vi "Read UDP.vi"(8 "error in (no error)":errorcluster, 11 "Telnet V2 in":refnum<class "Telnet V2.lvclass">) -> (0 "error out":errorcluster, 2 "String":string, 3 "Telnet V2 out":refnum<class "Telnet V2.lvclass">)   [LabVIEW 2018, in "Telnet V2.lvlib" / "Telnet V2.lvclass"]
uses:
  Telnet V2.lvclass
  Telnet V2.lvclass/Telnet V2.ctl
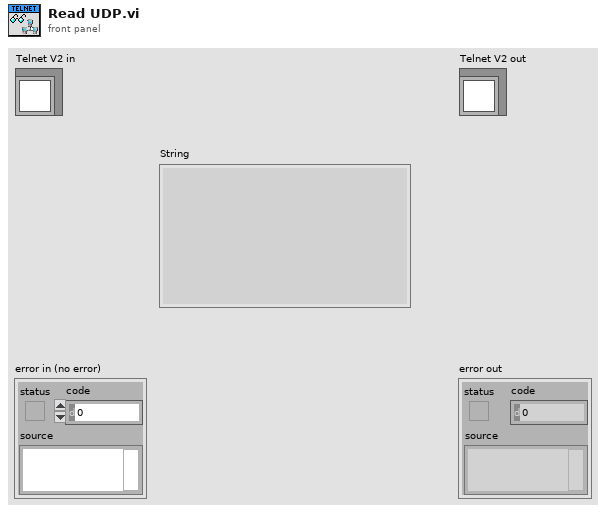
[diagram p1: front panel]
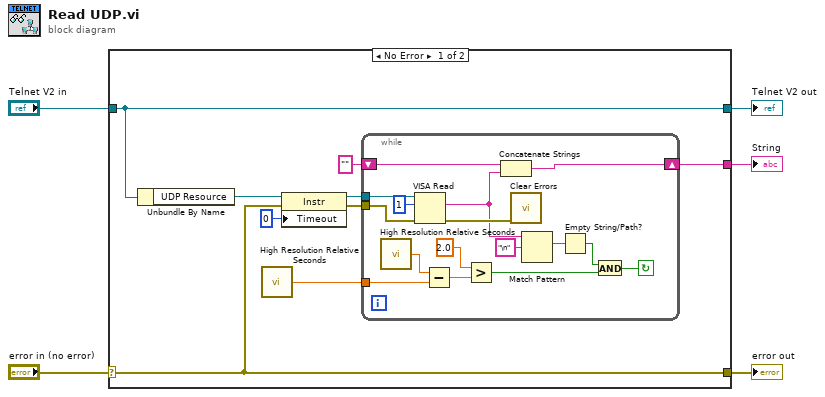
[diagram p0: block diagram]
diagram:
  n1 = case shown="No Error" "error in (no error)" {
    selector: "error in (no error)" -> [w7 w32]
    tunnel: [w7 w32] -> w4
    tunnel: [w8 w31] -> w2
    tunnel: "Telnet V2 in" -> [w8 w31]
    tunnel: [w6 _] -> w1
    frame No Error {
      n2 = Unbundle By Name(w8) -> ("UDP Resource"=w14:refnum<visa-resource-name>)
      n3 = call <vilib>:"High Resolution Relative Seconds.vi"() -> ("relative seconds"=w10:dbl)
      n4 = property class="Instr"(reference=w14, error in=w7, "Timeout"=u32 0 ("General Settings:Timeout Value")) -> (reference out=w13:refnum<visa-resource-name>, error out=w11:errorcluster)
      n5 = while {
        tunnel: w13 -> [w30]
        tunnel: w11 -> [w27]
        shift-right: [w26] -> w6
        shift-left: "" -> [w25]
        tunnel: w10 -> [w23]
        stop <- w15 continue-if-true
        n6 = call <vilib>:"High Resolution Relative Seconds.vi"() -> ("relative seconds"=w24:dbl)
        n7 = VISA Read(VISA resource name=w30, byte count=u32 1, error in (no error)=w27) -> (read buffer=w20:string, error out=w28:errorcluster)  [unwired: 2 out]
        n8 = Subtract(x=w24, y=w23) -> (x-y=w21:dbl)
        n9 = Greater?(x=2.0, y=w21) -> (0:w16:bool)
        n10 = Concatenate Strings(w25, w20) -> (w26:string)
        n11 = call <vilib>:"Clear Errors.vi"("error in (no error)"=w28) -> ()  [unwired: 5 in, 2 out]
        n12 = Match Pattern(string=w20, regular expression="\n") -> (match substring=w18:string)  [unwired: 1 in, 3 out]
        n13 = Empty String/Path?(string/path=w18) -> (empty?=w17:bool)
        n14 = And(x=w17, y=w16) -> (x .and. y?=w15:bool)
      }
    }
    frame Error {
    }
  }
  "error out" <- w4
  "Telnet V2 out" <- w2
  "String" <- w1
